vi "Normalise_profile.vi"() -> (0 "New Values In":string[][](array[string])=[["Test data5"]], 1 "New Chs In":string[](array[string])=["30-10-03:New:Channel new5"])   [LabVIEW 2020]
uses:
  Results_plotter_Global.vi
  <vilib>/Analysis/NI_AALBase.lvlib
  Data plotting/subVIs/Plot_Values_Global.vi
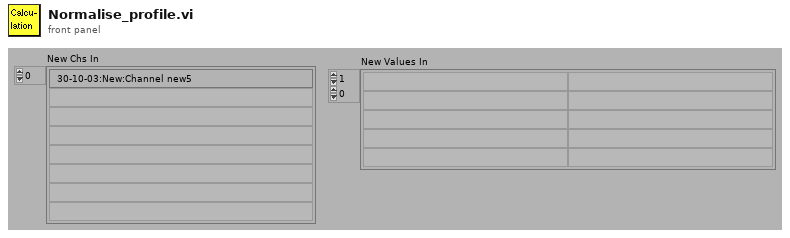
[diagram p1: front panel]
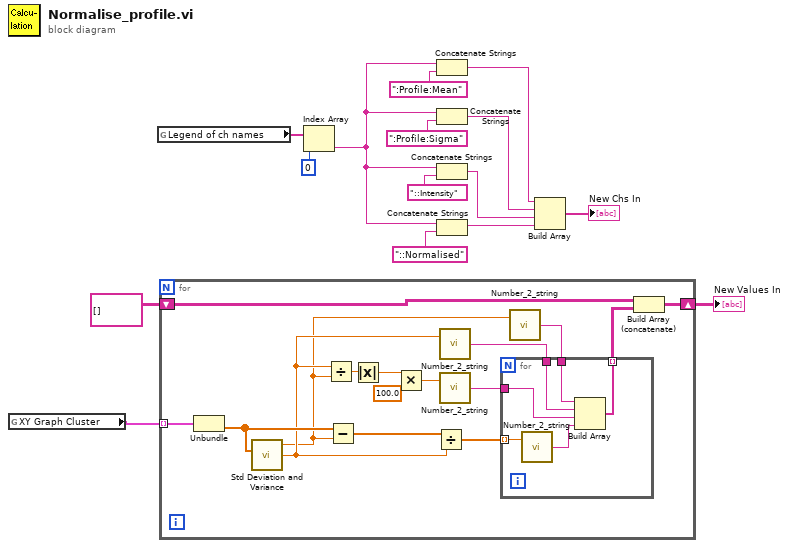
[diagram p0: block diagram]
diagram:
  n1 = global read "Plot_Values_Global.vi" "XY Graph Cluster"() -> (w1:cluster{dbl[], dbl[]}[])
  n2 = global read "Results_plotter_Global.vi" "Legend of ch names"() -> (w12:string[])
  n3 = for {
    tunnel: w1 -> [w31] mode=indexing
    shift-right: [w24] -> w8
    shift-left: string[][] [] -> [w28]
    n4 = Unbundle(w31) -> (w30:dbl[])  [unwired: 1 out]
    n5 = call <vilib>:"Std Deviation and Variance.vi"("X"=w30) -> ("mean"=w17:dbl, "standard deviation"=w19:dbl)  [unwired: 1 in, 1 out]
    n6 = Divide(x=w19, y=w17) -> (x/y=w23:dbl)
    n7 = Subtract(x=w30, y=w17) -> (x-y=w29:dbl[])
    n8 = Absolute Value(x=w23) -> (abs(x)=w22:dbl)
    n9 = Multiply(x=w22, y=100.0) -> (x*y=w20:dbl)
    n10 = Divide(x=w29, y=w19) -> (x/y=w27:dbl[])
    n11 = call "Number_2_string.vi"("number"=w19) -> ("String"=w18:string)  [unwired: 1 in]
    n12 = call "Number_2_string.vi"("number"=w20) -> ("String"=w26:string)  [unwired: 1 in]
    n13 = call "Number_2_string.vi"("number"=w17) -> ("String"=w16:string)  [unwired: 1 in]
    n14 = for {
      tunnel: w27 -> [w37] mode=indexing
      tunnel: w26 -> [w35]
      tunnel: [w34] -> w25 mode=indexing
      tunnel: w18 -> [w33]
      tunnel: w16 -> [w32]
      n15 = call "Number_2_string.vi"("number"=w37) -> ("String"=w36:string)  [unwired: 1 in]
      n16 = Build Array(w32, w33, w35, w36) -> (w34:string[])
    }
    n17 = Build Array (concatenate)(w28, w25) -> (w24:string[][])
  }
  "New Values In" <- w8
  n18 = Index Array(array=w12, index=0) -> (element=w3:string)
  n19 = Concatenate Strings(w3, ":Profile:Mean" ("string")) -> (w2:string)
  n20 = Concatenate Strings(w3, ":Profile:Sigma" ("string")) -> (w5:string)
  n21 = Concatenate Strings(w3, "::Intensity" ("string")) -> (w10:string)
  n22 = Concatenate Strings(w3, "::Normalised" ("string")) -> (w9:string)
  n23 = Build Array(w2, w5, w10, w9) -> (→"New Chs In":string[])
